vi "Uint8 Destroy.vi"(8 "error in (no error)":errorcluster, 11 "Uint8 DVR in":refnum<data-value>) -> (0 "error out":errorcluster)   [LabVIEW 2010, in "MDSplus.lvlib"]
uses:
  <vilib>/MDSplus/Library/MDSplus.lvlib
  <vilib>/MDSplus/Classes/Data_Class/Scalar_Class/Uint8_Class/Uint8.lvclass
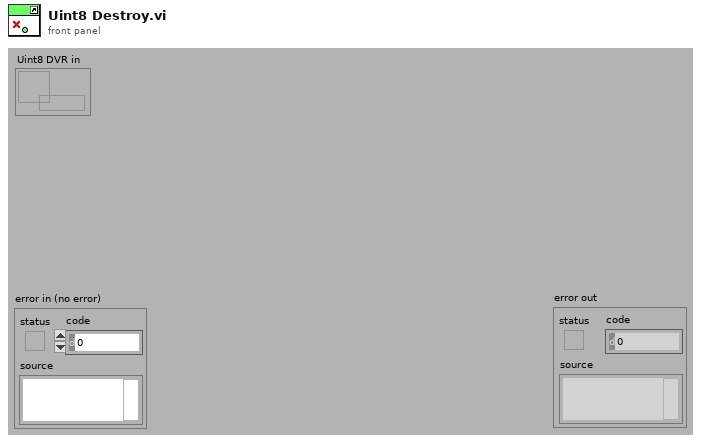
[diagram p1: front panel]
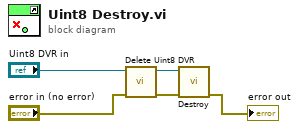
[diagram p0: block diagram]
diagram:
  n1 = call <vilib>:"Delete Uint8 DVR.vi"("error in (no error)"="error in (no error)", "Uint8 DVR in"="Uint8 DVR in") -> ("error out"=w2:errorcluster, "Uint8 out"=w3:refnum<class "Uint8.lvclass">)  [unwired: 8 in]
  n2 = call-dynamic "Destroy.vi"("error in (no error)"=w2, "Uint8 in"=w3) -> ("error out"=→"error out":errorcluster)  [unwired: 9 in]
